vi "Scale Channels.vi"(5 "Scaling Classes":refnum<class "Scaling.lvclass">[](array[class]), 7 "Used Scalings":string[](array[string]), 8 "error in (no error)":errorcluster, 9 "Channel Names":string[](array[string]), 10 "Values In":dbl[](array[numeric]), 11 "Scaling in":refnum<class "Scaling.lvclass">) -> (0 "error out":errorcluster, 2 "Values Out":dbl[](array[numeric]), 3 "Scaling out":refnum<class "Scaling.lvclass">)   [LabVIEW 2024, in "Scaling.lvclass"]
doc: "Scaling.lvclass:Scale Channels.vi\n\nThis is the template for the Scale Channels VI forthe Scaling class.\n\nInstrument Communication Module Version 1.0\nSeptember, 2017 Original Code Consulting David Thomson\n www.originalcode.com"
uses:
  Scaling.lvclass
  Scaling.lvclass/Scaling.ctl
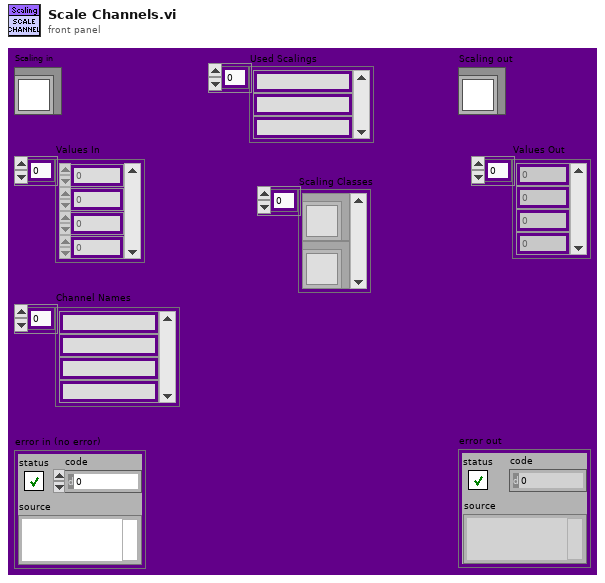
[diagram p1: front panel]
types:
  T1 = typedef "Scaling Def.ctl" = cluster{"Channel":string, "Scaling":string, "Instance":string}
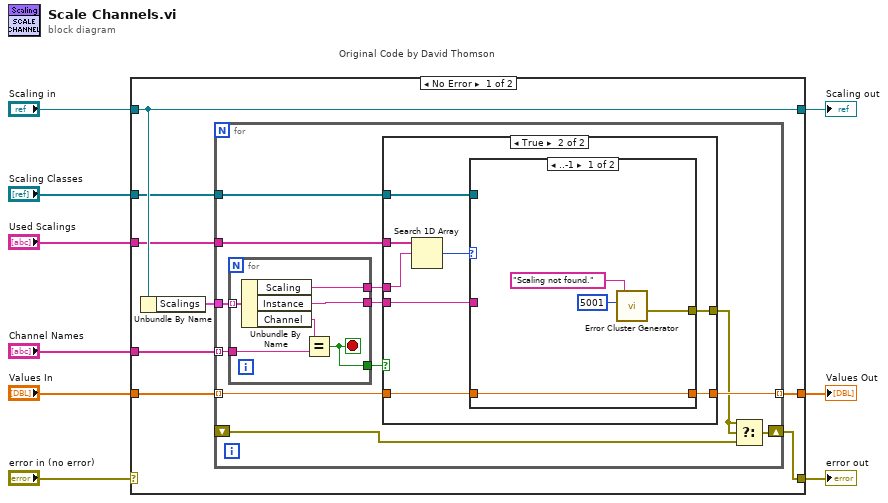
[diagram p0: block diagram]
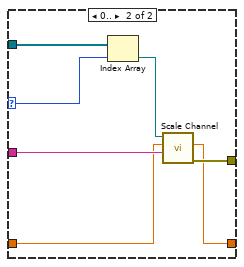
[diagram p3: hidden frame]
diagram:
  n1 = case "Original Code by David Thomson" shown="No Error" "error in (no error)" {
    selector: "error in (no error)" -> [_ w58]
    tunnel: [w13 w58] -> w8
    tunnel: [w12 w57] -> w6
    tunnel: "Scaling in" -> [w12 w57]
    tunnel: "Values In" -> [w17 w56]
    tunnel: "Channel Names" -> [w16 _]
    tunnel: [w14 w56] -> w3
    tunnel: "Scaling Classes" -> [w11 _]
    tunnel: "Used Scalings" -> [w10 _]
    frame No Error {
      n2 = Unbundle By Name(w12) -> ("Scalings"=w15:T1[])
      n3 = for {
        tunnel: w17 -> [w25] mode=indexing
        tunnel: w16 -> [w28] mode=indexing
        tunnel: w15 -> [w29]
        tunnel: [w26] -> w14 mode=indexing
        shift-right: [w21] -> w13
        shift-left: _ -> [w22]
        tunnel: w11 -> [w18]
        tunnel: w10 -> [w19]
        n4 = for {
          tunnel: w29 -> [w55] mode=indexing
          tunnel: w28 -> [w53]
          tunnel: [w52] -> w27
          tunnel: [w51] -> w24
          tunnel: [w50] -> w23
          stop <- w52 stop-if-true
          n5 = Unbundle By Name(w55) -> ("Scaling"=w51:string, "Instance"=w50:string, "Channel"=w54:string)
          n6 = Equal?(x=w54, y=w53) -> (x = y?=w52:bool)
        }
        n7 = case shown="True" w27 {
          tunnel: [w30 w36] -> w26
          tunnel: w25 -> [w30 w38]
          tunnel: w24 -> [_ w33]
          tunnel: w23 -> [_ w35]
          tunnel: [_ w37] -> w20
          tunnel: w19 -> [_ w34]
          tunnel: w18 -> [_ w32]
          frame False {
          }
          frame True {
            n8 = Search 1D Array(1D array=w34, element=w33) -> (index of element=w31:i32)  [unwired: 1 in]
            n9 = case shown="..-1" w31 {
              selector: w31 -> [_ w45]
              tunnel: w38 -> [w42 w44]
              tunnel: [w41 w49] -> w37
              tunnel: [w42 w43] -> w36
              tunnel: w35 -> [_ w48]
              tunnel: w32 -> [_ w47]
              frame ..-1 {
                n10 = call "Error Cluster Generator.vi"("code"=5001, "Additional message"="Scaling not found.") -> ("error out"=w41:errorcluster)  [unwired: 4 in, 1 out]
              }
              frame 0.. {
                n11 = Index Array(array=w47, index=w45) -> (element=w46:refnum<class "Scaling.lvclass">)
                n12 = call-dynamic "Scale Channel.vi"("Instance"=w48, "Value In"=w44, "Scaling in"=w46) -> ("error out"=w49:errorcluster, "Value Out"=w43:dbl)  [unwired: 6 in, 1 out]
              }
            }
          }
        }
        n13 = Select(t=w20, s=w20, f=w22) -> (s? t:f=w21:errorcluster)
      }
    }
    frame Error {
    }
  }
  "error out" <- w8
  "Scaling out" <- w6
  "Values Out" <- w3
